vi "test_Create Message_Existing Message Name Error.vi"(8 "error in (no error)":errorcluster, 11 "TestCase in":refnum<class "Instrument Addon Scripting API Messages Unit Tests.lvclass">) -> (0 "error out":errorcluster, 3 "TestCase out":refnum<class "Instrument Addon Scripting API Messages Unit Tests.lvclass">)   [LabVIEW 2023, in "Instrument Addon Scripting API Messages Unit Tests.lvclass"]
uses:
  Instrument Addon Scripting API Messages Unit Tests.lvclass
  Instrument Addon Scripting API Messages Unit Tests.lvclass/Instrument Addon Scripting API Messages Unit Tests.ctl
  <vilib>/addons/_JKI Toolkits/VI Tester/TestCase.llb/TestCase.lvclass
  APIs/Scripting API/Instrument Addon Scripting API.lvlib
  NationalInstruments.VeriStand.SystemDefinitionAPI
  <vilib>/NI VeriStand/Custom Device Tools/Custom Device Utility Library/Custom Device Utility Library.lvlib
  Addon/Addon Shared/SubVIs/Constants.vi
  Addon/Addon Shared/Instrument Addon Shared.lvlib
  APIs/Scripting API/TypeDefs/Protection Types.ctl
  APIs/Scripting API/TypeDefs/Message Settings.ctl
  <vilib>/NI VeriStand/Custom Device Tools/Custom Device Utility Library/NI VeriStand - Search for Item by GUID.vi
  APIs/Scripting API/Messages/Create Message - Trigger Only.vi
  C:/Program Files (x86)/National Instruments/LabVIEW 2020/vi.lib/addons/_JKI Toolkits/VI Tester/TestCase.llb/TestCase.lvclass
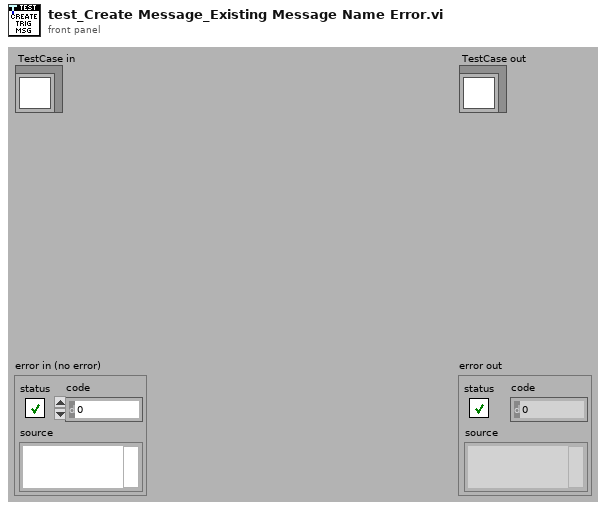
[diagram p1: front panel]
types:
  T1 = typedef "Instrument Addon Scripting API.lvlib/Message Settings.ctl" = cluster{"Protection":T2, "Enable Periodic Default":bool, "Trigger Channel refnum":u64}
  T2 = typedef "Instrument Addon Scripting API.lvlib/Protection Types.ctl" = enum16{"None", "CRC-32", "Checksum U16", "Checksum U32", "Checksum U8"}
  T3 = typedef "Custom Device API.lvlib/Custom Device Item Ref.ctl" = u64
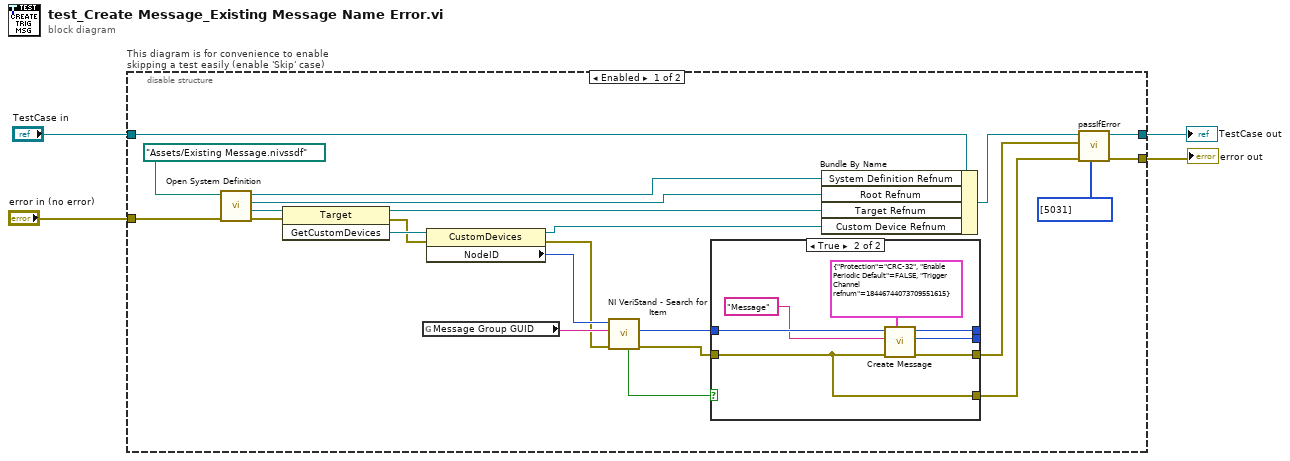
[diagram p0: block diagram]
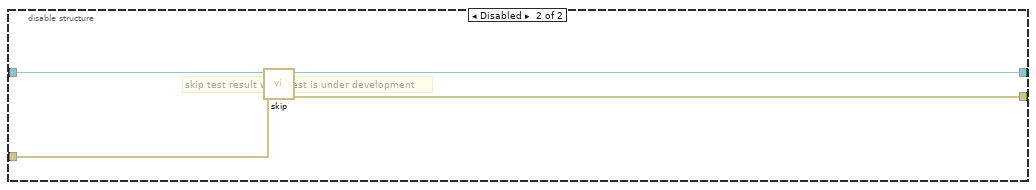
[diagram p3: hidden frame]
diagram:
  n1 = disable-structure "This diagram is for convenience to enable skipping a test easily (enable 'Skip' case)" shown="Enabled" {
    disable-tunnel: "TestCase in" -> [w13 w39]
    disable-tunnel: [w14 w37] -> w1
    disable-tunnel: [w15 w38] -> w3
    disable-tunnel: "error in (no error)" -> [w26 w36]
    frame Enabled {
      n2 = call "Open System Definition.vi"("error in (no error)"=w26, "System Definition File"=path "Assets/Existing Message.nivssdf" ("SDF file")) -> ("error out"=w19:errorcluster, "Target Refnum"=w25:refnum<k24>, "Root Refnum"=w11:refnum<k24>, "System Definition Refnum"=w12:refnum<k24>)  [unwired: 6 in]
      n3 = invoke class="Target" method="GetCustomDevices"(reference=w25, error in=w19) -> (reference out=w10:refnum<k24>, error out=w18:errorcluster, "GetCustomDevices"=w24:refnum<k24>)  [unwired: 1 in]
      n4 = global read "Constants.vi" "Message Group GUID"() -> (w22:string)
      n5 = property class="CustomDevices"(reference=w24, error in=w18) -> (reference out=w8:refnum<k24>, error out=w17:errorcluster, "NodeID"=w23:u64)
      n6 = call-poly <vilib>:"NI VeriStand - Search for Item.vi"("error in"=w17, "Item GUID"=w22, "Section Ref in"=w23) -> ("error out"=w16:errorcluster, "Item Ref"=w21:T3, "Found"=w20:bool)  [unwired: 5 in, 1 out]
      n7 = case shown="True" w20 {
        tunnel: w21 -> [_ w35]
        tunnel: [w28 w34] -> w6
        tunnel: w16 -> [w28 w30]
        tunnel: [_ w33] -> _
        tunnel: [_ w32] -> _
        tunnel: [_ w30] -> w7
        frame False {
        }
        frame True {
          n8 = call-poly "Create Message.vi"("optional settings"=T1 {"Protection"=enum."CRC-32", "Enable Periodic Default"=FALSE, "Trigger Channel refnum"=18446744073709551615} ("Message Settings"), "error in (no error)"=w30, "message name"="Message", "message group refnum in"=w35) -> ("error out"=w34:errorcluster, "message refnum out"=w33:T3, "message group refnum out"=w32:T3)  [unwired: 5 in]
        }
      }
      n9 = Bundle By Name(cluster=w13, "System Definition Refnum"=w12, "Root Refnum"=w11, "Target Refnum"=w10, "Custom Device Refnum"=w8) -> (w9:refnum<class "Instrument Addon Scripting API Messages Unit Tests.lvclass">)
      n10 = call-dynamic "passIfError.vi"("passing error codes (default = any error code)"=i32[] [5031], "error in (no error)"=w7, "error"=w6, "TestCase in"=w9) -> ("error out"=w15:errorcluster, "TestCase out"=w14:refnum<class "Instrument Addon Scripting API Messages Unit Tests.lvclass">)  [unwired: 6 in]
    }
    frame Disabled {
      # "skip test result while test is under development"
      n11 = call <vilib>:"skip.vi"("error in (no error)"=w36, "TestCase in"=w39) -> ("error out"=w38:errorcluster, "TestCase out"=w37:refnum<class "Instrument Addon Scripting API Messages Unit Tests.lvclass">)  [unwired: 8 in]
    }
  }
  "error out" <- w3
  "TestCase out" <- w1
